vi "ReadRecipe.vi"(5 "RcpFilePath":path) -> (0 "Success":bool, 1 "TestPara":T3={"LoadType"=enum."15kW伺服馬達", "DegSetValue"=0.0, "LoadSideWave"={"TestSpeed"=0.0, "Crest"=0.0, "Trugh"=0.0, "TestTorque"=0.0}, "DriveSideWave"={"TestSpeed"=0.0, "LoadValue"=0.0, "Crest"=0.0, "Trugh"=0.0}, "MultiPt"={"Program_Multi"=[], "InitSpeed"=0.0, "PID"={"NP"=0.0, "NI"=0.0, "ND"=0.0, "NPS"="A", "NIS"="A", "NDS"="A"}, "TestTorque"=0.0}, "MultiPtStall"={"Program_Multi"=[], "InitSpeed"=0.0, "PID"={"NP"=0.0, "NI"=0.0, "ND"=0.0, "NPS"="A", "NIS"="A", "NDS"="A"}, "LoadValue"=0.0}, "FixPt"={"InitSpeed"=0.0, "PID"={"NP"=0.0, "NI"=0.0, "ND"=0.0, "NPS"="A", "NIS"="A", "NDS"="A"}, "LoadValue"=0.0, "TestTorque"=0.0}, "FixPtStall"={"InitSpeed"=0.0, "PID"={"NP"=0.0, "NI"=0.0, "ND"=0.0, "NPS"="A", "NIS"="A", "NDS"="A"}, "LoadValue"=0.0}} {"FixPtStall"."LoadValue" format="%#_2f"; "FixPtStall"."PID"."ND" min=0.0 max=99.0 format="%#.2f"; "FixPtStall"."PID"."NI" min=0.0 max=99.0 step=1.0 format="%#.2f"; "FixPtStall"."PID"."NP" min=0.0 max=99.0 format="%#.2f"; "FixPtStall"."InitSpeed" format="%#_2f"; "FixPt"."TestTorque" format="%#_2f"; "FixPt"."LoadValue" min=0.0 max=99.0 format="%#.2f"; "FixPt"."PID"."ND" min=0.0 max=99.0 format="%#.2f"; "FixPt"."PID"."NI" min=0.0 max=99.0 step=1.0 format="%#.2f"; "FixPt"."PID"."NP" min=0.0 max=99.0 format="%#.2f"; "FixPt"."InitSpeed" min=0.0 max=99.0 format="%#.2f"; "MultiPtStall"."LoadValue" format="%#_2f"; "MultiPtStall"."PID"."ND" min=0.0 max=99.0 format="%#.2f"; "MultiPtStall"."PID"."NI" min=0.0 max=99.0 step=1.0 format="%#.2f"; "MultiPtStall"."PID"."NP" min=0.0 max=99.0 format="%#.2f"; "MultiPtStall"."InitSpeed" format="%#_2f"; "MultiPt"."TestTorque" format="%#_2f"; "MultiPt"."PID"."ND" min=0.0 max=99.0 format="%#.2f"; "MultiPt"."PID"."NI" min=0.0 max=99.0 step=1.0 format="%#.2f"; "MultiPt"."PID"."NP" min=0.0 max=99.0 format="%#.2f"; "MultiPt"."InitSpeed" format="%#_2f"; "DriveSideWave"."Trugh" format="%#_2f"; "DriveSideWave"."Crest" format="%#_2f"; "DriveSideWave"."LoadValue" format="%#_2f"; "DriveSideWave"."TestSpeed" format="%#_2f"; "LoadSideWave"."TestTorque" format="%#_2f"; "LoadSideWave"."Trugh" format="%#_2f"; "LoadSideWave"."Crest" format="%#_2f"; "LoadSideWave"."TestSpeed" format="%#_2f"}, 2 "RcpFilePath.dup":path)   [LabVIEW 2024]
uses:
  MFActor/TestParameter.ctl
panel:
  in  "TestPara_V2":T1={"LoadType"=enum."15kW伺服馬達", "DegSetValue"=0.0, "LoadSideWave"={"TestSpeed"=0.0, "Crest"=0.0, "Trugh"=0.0, "TestTorque"=0.0}, "DriveSideWave"={"TestSpeed"=0.0, "LoadValue"=0.0, "Crest"=0.0, "Trugh"=0.0}, "MultiPt"={"Program_Multi"=[], "InitSpeed"=0.0, "PID"={"NP"=0.0, "NI"=0.0, "ND"=0.0, "NPS"="A", "NIS"="A", "NDS"="A"}, "TestTorque"=0.0}, "MultiPtStall"={"Program_Multi"=[], "InitSpeed"=0.0, "PID"={"NP"=0.0, "NI"=0.0, "ND"=0.0, "NPS"="A", "NIS"="A", "NDS"="A"}, "LoadValue"=0.0}, "FixPt"={"InitSpeed"=0.0, "PID"={"NP"=0.0, "NI"=0.0, "ND"=0.0, "NPS"="A", "NIS"="A", "NDS"="A"}, "LoadValue"=0.0, "TestTorque"=0.0}, "FixPtStall"={"InitSpeed"=0.0, "PID"={"NP"=0.0, "NI"=0.0, "ND"=0.0, "NPS"="A", "NIS"="A", "NDS"="A"}, "LoadValue"=0.0}} {"FixPtStall"."LoadValue" format="%#_2f"; "FixPtStall"."PID"."ND" min=0.0 max=99.0 format="%#.2f"; "FixPtStall"."PID"."NI" min=0.0 max=99.0 step=1.0 format="%#.2f"; "FixPtStall"."PID"."NP" min=0.0 max=99.0 format="%#.2f"; "FixPtStall"."InitSpeed" format="%#_2f"; "FixPt"."TestTorque" format="%#_2f"; "FixPt"."LoadValue" format="%#_2f"; "FixPt"."PID"."ND" min=0.0 max=99.0 format="%#.2f"; "FixPt"."PID"."NI" min=0.0 max=99.0 step=1.0 format="%#.2f"; "FixPt"."PID"."NP" min=0.0 max=99.0 format="%#.2f"; "FixPt"."InitSpeed" format="%#_2f"; "MultiPtStall"."LoadValue" format="%#_2f"; "MultiPtStall"."PID"."ND" min=0.0 max=99.0 format="%#.2f"; "MultiPtStall"."PID"."NI" min=0.0 max=99.0 step=1.0 format="%#.2f"; "MultiPtStall"."PID"."NP" min=0.0 max=99.0 format="%#.2f"; "MultiPtStall"."InitSpeed" format="%#_2f"; "MultiPt"."TestTorque" format="%#_2f"; "MultiPt"."PID"."ND" min=0.0 max=99.0 format="%#.2f"; "MultiPt"."PID"."NI" min=0.0 max=99.0 step=1.0 format="%#.2f"; "MultiPt"."PID"."NP" min=0.0 max=99.0 format="%#.2f"; "MultiPt"."InitSpeed" format="%#_2f"; "DriveSideWave"."Trugh" format="%#_2f"; "DriveSideWave"."Crest" format="%#_2f"; "DriveSideWave"."LoadValue" format="%#_2f"; "DriveSideWave"."TestSpeed" format="%#_2f"; "LoadSideWave"."TestTorque" format="%#_2f"; "LoadSideWave"."Trugh" format="%#_2f"; "LoadSideWave"."Crest" format="%#_2f"; "LoadSideWave"."TestSpeed" format="%#_2f"}
  in  "TestPara_V1":T2={"LoadType"=enum."15kW伺服馬達", "DegSetValue"=0.0, "LoadSideWave"={"TestSpeed"=0.0, "Crest"=0.0, "Trugh"=0.0}, "DriveSideWave"={"TestSpeed"=0.0, "LoadValue"=0.0, "Crest"=0.0, "Trugh"=0.0}, "MultiPt"={"Program_Multi"=[], "InitSpeed"=0.0, "PID"={"NP"=0.0, "NI"=0.0, "ND"=0.0, "NPS"="A", "NIS"="A", "NDS"="A"}}, "MultiPtStall"={"Program_Multi"=[], "InitSpeed"=0.0, "PID"={"NP"=0.0, "NI"=0.0, "ND"=0.0, "NPS"="A", "NIS"="A", "NDS"="A"}, "LoadValue"=0.0}, "FixPt"={"InitSpeed"=0.0, "PID"={"NP"=0.0, "NI"=0.0, "ND"=0.0, "NPS"="A", "NIS"="A", "NDS"="A"}, "LoadValue"=0.0}, "FixPtStall"={"InitSpeed"=0.0, "PID"={"NP"=0.0, "NI"=0.0, "ND"=0.0, "NPS"="A", "NIS"="A", "NDS"="A"}, "LoadValue"=0.0}} {"FixPtStall"."LoadValue" format="%#_2f"; "FixPtStall"."PID"."ND" min=0.0 max=99.0 format="%#.2f"; "FixPtStall"."PID"."NI" min=0.0 max=99.0 step=1.0 format="%#.2f"; "FixPtStall"."PID"."NP" min=0.0 max=99.0 format="%#.2f"; "FixPtStall"."InitSpeed" format="%#_2f"; "FixPt"."LoadValue" format="%#_2f"; "FixPt"."PID"."ND" min=0.0 max=99.0 format="%#.2f"; "FixPt"."PID"."NI" min=0.0 max=99.0 step=1.0 format="%#.2f"; "FixPt"."PID"."NP" min=0.0 max=99.0 format="%#.2f"; "FixPt"."InitSpeed" format="%#_2f"; "MultiPtStall"."LoadValue" format="%#_2f"; "MultiPtStall"."PID"."ND" min=0.0 max=99.0 format="%#.2f"; "MultiPtStall"."PID"."NI" min=0.0 max=99.0 step=1.0 format="%#.2f"; "MultiPtStall"."PID"."NP" min=0.0 max=99.0 format="%#.2f"; "MultiPtStall"."InitSpeed" format="%#_2f"; "MultiPt"."PID"."ND" min=0.0 max=99.0 format="%#.2f"; "MultiPt"."PID"."NI" min=0.0 max=99.0 step=1.0 format="%#.2f"; "MultiPt"."PID"."NP" min=0.0 max=99.0 format="%#.2f"; "MultiPt"."InitSpeed" format="%#_2f"; "DriveSideWave"."Trugh" format="%#_2f"; "DriveSideWave"."Crest" format="%#_2f"; "DriveSideWave"."LoadValue" format="%#_2f"; "DriveSideWave"."TestSpeed" format="%#_2f"; "LoadSideWave"."Trugh" format="%#_2f"; "LoadSideWave"."Crest" format="%#_2f"; "LoadSideWave"."TestSpeed" format="%#_2f"}
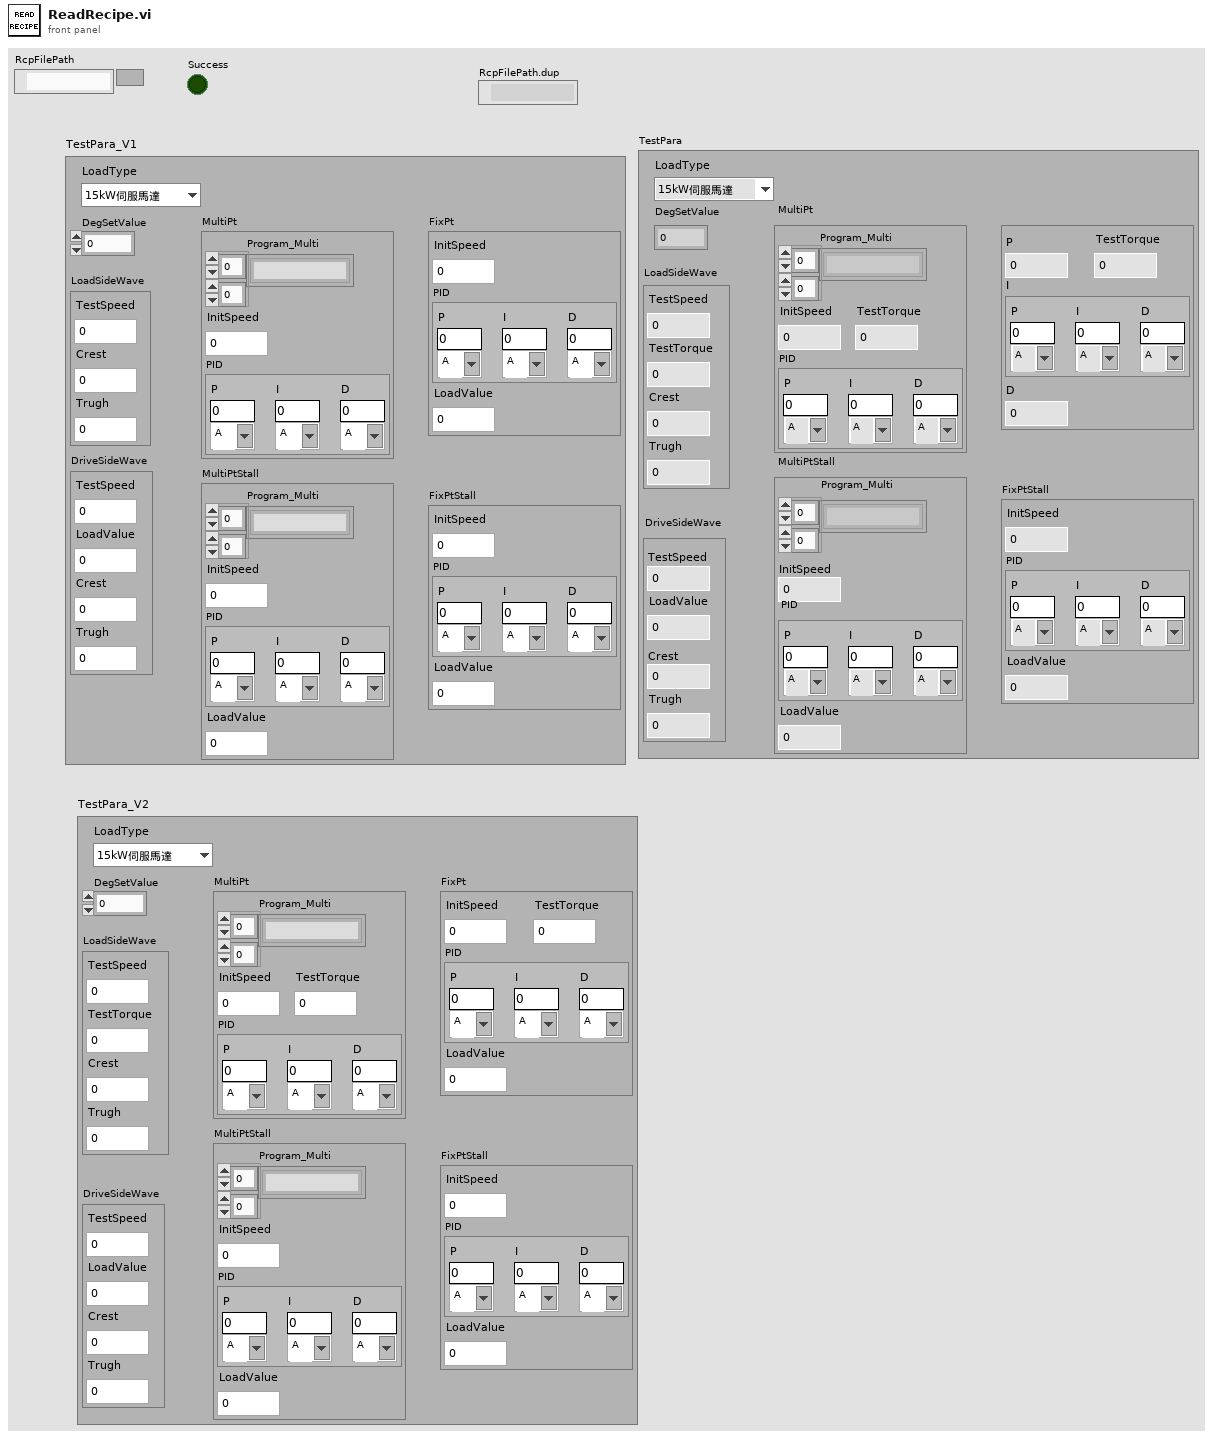
[diagram p1: front panel]
types:
  T1 = cluster{"LoadType":enum16{"15kW伺服馬達", "煞車器"}, "DegSetValue":dbl, "LoadSideWave":cluster{"TestSpeed":dbl, "Crest":dbl, "Trugh":dbl, "TestTorque":dbl}, "DriveSideWave":cluster{"TestSpeed":dbl, "LoadValue":dbl, "Crest":dbl, "Trugh":dbl}, "MultiPt":cluster{"Program_Multi":string[][], "InitSpeed":dbl, "PID":cluster{"NP":dbl, "NI":dbl, "ND":dbl, "NPS":string, "NIS":string, "NDS":string}, "TestTorque":dbl}, "MultiPtStall":cluster{"Program_Multi":string[][], "InitSpeed":dbl, "PID":cluster{"NP":dbl, "NI":dbl, "ND":dbl, "NPS":string, "NIS":string, "NDS":string}, "LoadValue":dbl}, "FixPt":cluster{"InitSpeed":dbl, "PID":cluster{"NP":dbl, "NI":dbl, "ND":dbl, "NPS":string, "NIS":string, "NDS":string}, "LoadValue":dbl, "TestTorque":dbl}, "FixPtStall":cluster{"InitSpeed":dbl, "PID":cluster{"NP":dbl, "NI":dbl, "ND":dbl, "NPS":string, "NIS":string, "NDS":string}, "LoadValue":dbl}}
  T2 = cluster{"LoadType":enum16{"15kW伺服馬達", "煞車器"}, "DegSetValue":dbl, "LoadSideWave":cluster{"TestSpeed":dbl, "Crest":dbl, "Trugh":dbl}, "DriveSideWave":cluster{"TestSpeed":dbl, "LoadValue":dbl, "Crest":dbl, "Trugh":dbl}, "MultiPt":cluster{"Program_Multi":string[][], "InitSpeed":dbl, "PID":cluster{"NP":dbl, "NI":dbl, "ND":dbl, "NPS":string, "NIS":string, "NDS":string}}, "MultiPtStall":cluster{"Program_Multi":string[][], "InitSpeed":dbl, "PID":cluster{"NP":dbl, "NI":dbl, "ND":dbl, "NPS":string, "NIS":string, "NDS":string}, "LoadValue":dbl}, "FixPt":cluster{"InitSpeed":dbl, "PID":cluster{"NP":dbl, "NI":dbl, "ND":dbl, "NPS":string, "NIS":string, "NDS":string}, "LoadValue":dbl}, "FixPtStall":cluster{"InitSpeed":dbl, "PID":cluster{"NP":dbl, "NI":dbl, "ND":dbl, "NPS":string, "NIS":string, "NDS":string}, "LoadValue":dbl}}
  T3 = typedef "TestParameter.ctl" = cluster{"LoadType":enum16{"15kW伺服馬達", "煞車器"}, "DegSetValue":dbl, "LoadSideWave":cluster{"TestSpeed":dbl, "Crest":dbl, "Trugh":dbl, "TestTorque":dbl}, "DriveSideWave":cluster{"TestSpeed":dbl, "LoadValue":dbl, "Crest":dbl, "Trugh":dbl}, "MultiPt":cluster{"Program_Multi":string[][], "InitSpeed":dbl, "PID":cluster{"NP":dbl, "NI":dbl, "ND":dbl, "NPS":string, "NIS":string, "NDS":string}, "TestTorque":dbl}, "MultiPtStall":cluster{"Program_Multi":string[][], "InitSpeed":dbl, "PID":cluster{"NP":dbl, "NI":dbl, "ND":dbl, "NPS":string, "NIS":string, "NDS":string}, "LoadValue":dbl}, "FixPt":cluster{"InitSpeed":dbl, "PID":cluster{"NP":dbl, "NI":dbl, "ND":dbl, "NPS":string, "NIS":string, "NDS":string}, "LoadValue":dbl, "TestTorque":dbl}, "FixPtStall":cluster{"InitSpeed":dbl, "PID":cluster{"NP":dbl, "NI":dbl, "ND":dbl, "NPS":string, "NIS":string, "NDS":string}, "LoadValue":dbl}}
  T4 = enum16{"open", "replace", "create", "open or create", "replace or create", "replace or create with confirmation"}
  T5 = cluster{"InitSpeed":dbl, "PID":cluster{"NP":dbl, "NI":dbl, "ND":dbl, "NPS":string, "NIS":string, "NDS":string}, "LoadValue":dbl, "TestTorque":dbl}
  T6 = cluster{"Program_Multi":string[][], "InitSpeed":dbl, "PID":cluster{"NP":dbl, "NI":dbl, "ND":dbl, "NPS":string, "NIS":string, "NDS":string}, "TestTorque":dbl}
  T7 = cluster{"TestSpeed":dbl, "Crest":dbl, "Trugh":dbl, "TestTorque":dbl}
  T8 = cluster{"TestSpeed":dbl, "Crest":dbl, "Trugh":dbl}
  T9 = cluster{"TestSpeed":dbl, "LoadValue":dbl, "Crest":dbl, "Trugh":dbl}
  T10 = cluster{"Program_Multi":string[][], "InitSpeed":dbl, "PID":cluster{"NP":dbl, "NI":dbl, "ND":dbl, "NPS":string, "NIS":string, "NDS":string}}
  T11 = cluster{"Program_Multi":string[][], "InitSpeed":dbl, "PID":cluster{"NP":dbl, "NI":dbl, "ND":dbl, "NPS":string, "NIS":string, "NDS":string}, "LoadValue":dbl}
  T12 = cluster{"InitSpeed":dbl, "PID":cluster{"NP":dbl, "NI":dbl, "ND":dbl, "NPS":string, "NIS":string, "NDS":string}, "LoadValue":dbl}
  T13 = cluster{"NP":dbl, "NI":dbl, "ND":dbl, "NPS":string, "NIS":string, "NDS":string}
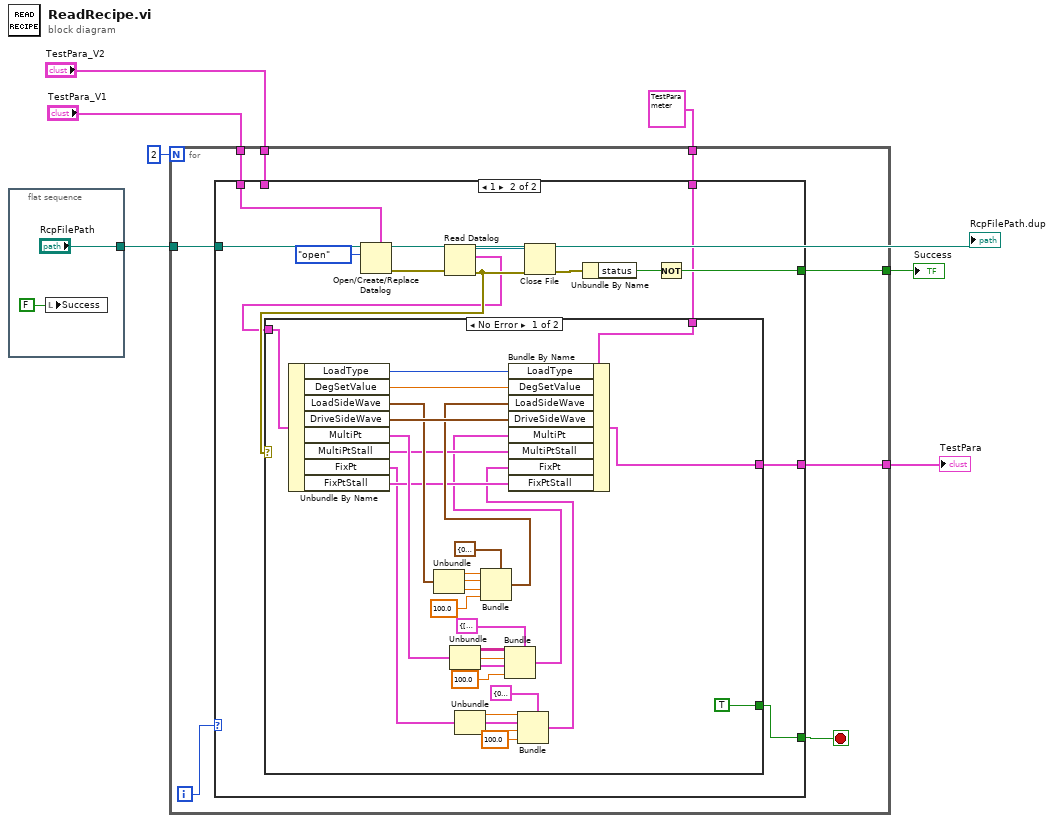
[diagram p0: block diagram]
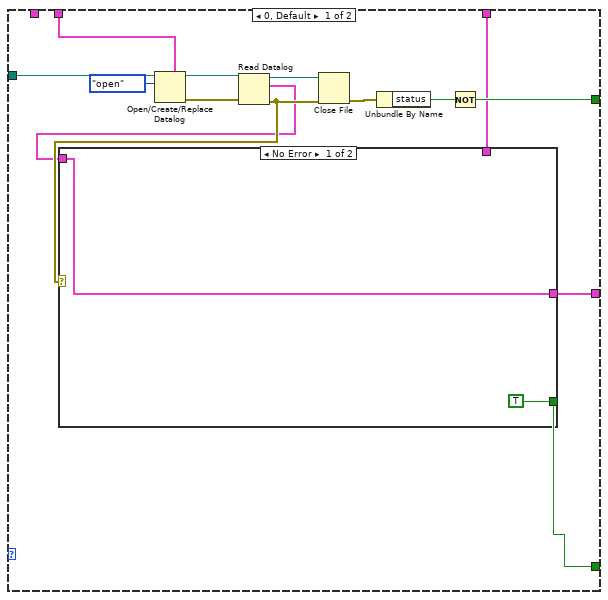
[diagram p2: hidden frame]
diagram:
  n1 = flat-sequence {
    tunnel: ["RcpFilePath"] -> w6
    frame #0 {
      n2 = local write "Success"(FALSE ("Success")) -> ()
    }
  }
  n3 = for {
    N: 2 -> [_]
    tunnel: w6 -> [w17]
    tunnel: "TestPara_V1" -> [w11]
    tunnel: [w15] -> w5
    tunnel: T3 {"LoadType"=enum."15kW伺服馬達", "DegSetValue"=0.0, "LoadSideWave"={"TestSpeed"=0.0, "Crest"=0.0, "Trugh"=0.0, "TestTorque"=0.0}, "DriveSideWave"={"TestSpeed"=0.0, "LoadValue"=0.0, "Crest"=0.0, "Trugh"=0.0}, "MultiPt"={"Program_Multi"=[], "InitSpeed"=0.0, "PID"={"NP"=0.0, "NI"=0.0, "ND"=0.0, "NPS"="A", "NIS"="A", "NDS"="A"}, "TestTorque"=0.0}, "MultiPtStall"={"Program_Multi"=[], "InitSpeed"=0.0, "PID"={"NP"=0.0, "NI"=0.0, "ND"=0.0, "NPS"="A", "NIS"="A", "NDS"="A"}, "LoadValue"=0.0}, "FixPt"={"InitSpeed"=0.0, "PID"={"NP"=0.0, "NI"=0.0, "ND"=0.0, "NPS"="A", "NIS"="A", "NDS"="A"}, "LoadValue"=0.0, "TestTorque"=0.0}, "FixPtStall"={"InitSpeed"=0.0, "PID"={"NP"=0.0, "NI"=0.0, "ND"=0.0, "NPS"="A", "NIS"="A", "NDS"="A"}, "LoadValue"=0.0}} ("TestPara") -> [w14]
    tunnel: [w13] -> w3
    tunnel: "TestPara_V2" -> [w10]
    i -> [w12]
    stop <- w16 stop-if-true
    n4 = case shown="1" w12 {
      tunnel: w17 -> [w27 w44]
      tunnel: w11 -> [_ w43]
      tunnel: [w26 w42] -> w16
      tunnel: [w23 w39] -> w15
      tunnel: w14 -> [w20 w36]
      tunnel: [w19 w35] -> w13
      tunnel: w10 -> [w18 _]
      frame 0, Default {
        n5 = Open/Create/Replace Datalog(5:w18, 10:T4."open" ("operation (0:open)"), 11:w27) -> (0:w30:errorcluster, 3:w29:refnum<k1>)  [unwired: 3 in, 1 out]
        n6 = Read Datalog(4:w30, 7:w29) -> (0:w22:errorcluster, 2:w21:T1, 3:w31:refnum<k1>)  [unwired: 1 in]
        n7 = case shown="No Error" w22 {
          tunnel: [TRUE _] -> w26
          tunnel: w21 -> [w32 _]
          tunnel: w20 -> [_ w34]
          tunnel: [w32 w34] -> w19
          frame No Error {
          }
          frame Error {
          }
        }
        n8 = Close File(refnum=w31, error in=w22) -> (error out=w25:errorcluster)  [unwired: 1 out]
        n9 = Unbundle By Name(w25) -> ("status"=w24:bool)
        n10 = Not(x=w24) -> (.not. x?=w23:bool)
      }
      frame 1 {
        n11 = Open/Create/Replace Datalog(5:w43, 10:T4."open" ("operation (0:open)"), 11:w44) -> (0:w47:errorcluster, 3:w46:refnum<k1>)  [unwired: 3 in, 1 out]
        n12 = Read Datalog(4:w47, 7:w46) -> (0:w38:errorcluster, 2:w37:T2, 3:w48:refnum<k1>)  [unwired: 1 in]
        n13 = case shown="No Error" w38 {
          tunnel: [TRUE _] -> w42
          tunnel: w37 -> [w77 _]
          tunnel: w36 -> [w76 w79]
          tunnel: [w49 w79] -> w35
          frame No Error {
            n14 = Unbundle By Name(w77) -> ("LoadType"=w75:enum16{"15kW伺服馬達", "煞車器"}, "DegSetValue"=w74:dbl, "LoadSideWave"=w72:T8, "DriveSideWave"=w73:T9, "MultiPt"=w65:T10, "MultiPtStall"=w64:T11, "FixPt"=w57:T12, "FixPtStall"=w58:T12)
            n15 = Unbundle(w72) -> ("TestSpeed"=w70:dbl, "Crest"=w69:dbl, "Trugh"=w68:dbl)
            n16 = Unbundle(w65) -> ("Program_Multi"=w62:string[][], "InitSpeed"=w61:dbl, "PID"=w60:T13)
            n17 = Unbundle(w57) -> ("InitSpeed"=w54:dbl, "PID"=w53:T13, "LoadValue"=w52:dbl)
            n18 = Bundle(cluster=T7 {"TestSpeed"=0.0, "Crest"=0.0, "Trugh"=0.0, "TestTorque"=0.0} ("LoadSideWave"), "TestSpeed"=w70, "Crest"=w69, "Trugh"=w68, "TestTorque"=100.0) -> (w66:T7)
            n19 = Bundle(cluster=T6 {"Program_Multi"=[], "InitSpeed"=0.0, "PID"={"NP"=0.0, "NI"=0.0, "ND"=0.0, "NPS"="", "NIS"="", "NDS"=""}, "TestTorque"=0.0} ("MultiPt"), "Program_Multi"=w62, "InitSpeed"=w61, "PID"=w60, "TestTorque"=100.0) -> (w56:T6)
            n20 = Bundle(cluster=T5 {"InitSpeed"=0.0, "PID"={"NP"=0.0, "NI"=0.0, "ND"=0.0, "NPS"="", "NIS"="", "NDS"=""}, "LoadValue"=0.0, "TestTorque"=0.0} ("FixPt"), "InitSpeed"=w54, "PID"=w53, "LoadValue"=w52, "TestTorque"=100.0) -> (w50:T5)
            n21 = Bundle By Name(cluster=w76, "LoadType"=w75, "DegSetValue"=w74, "LoadSideWave"=w66, "DriveSideWave"=w73, "MultiPt"=w56, "MultiPtStall"=w64, "FixPt"=w50, "FixPtStall"=w58) -> (w49:T3)
          }
          frame Error {
          }
        }
        n22 = Close File(refnum=w48, error in=w38) -> (error out=w41:errorcluster)  [unwired: 1 out]
        n23 = Unbundle By Name(w41) -> ("status"=w40:bool)
        n24 = Not(x=w40) -> (.not. x?=w39:bool)
      }
    }
  }
  "TestPara" <- w3
  "Success" <- w5
  "RcpFilePath.dup" <- w6
